vi "ConvertVoltToDegree1.vi"(10 "Tension":dbl[](array[numeric])) -> (2 "Température":dbl[](array[numeric]))   [LabVIEW 2018]
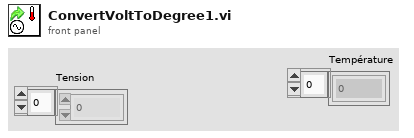
[diagram p1: front panel]
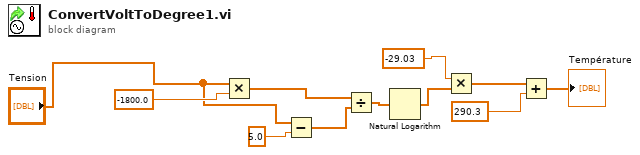
[diagram p0: block diagram]
diagram:
  n1 = Multiply(x="Tension", y=-1800.0) -> (x*y=w10:dbl[])
  n2 = Subtract(x="Tension", y=5.0 ("x")) -> (x-y=w1:dbl[])
  n3 = Divide(x=w10, y=w1) -> (x/y=w9:dbl[])
  n4 = Natural Logarithm(1:w9) -> (0:w8:dbl[])
  n5 = Multiply(x=-29.03, y=w8) -> (x*y=w7:dbl[])
  n6 = Add(x=w7, y=290.3 ("x")) -> (x+y=→"Température":dbl[])
